vi "Add Signal.vi"(8 "error in":errorcluster, 9 "Signal":refnum<class "CAN Signal.lvclass">, 10 "Signal Name":string, 11 "CAN Frame in":refnum<class "CAN Frame.lvclass">) -> (0 "error out":errorcluster, 3 "CAN Frame out":refnum<class "CAN Frame.lvclass">)   [LabVIEW 2023, in "CAN Frame.lvclass"]
uses:
  CAN Frame.lvclass
  CAN Frame.lvclass/CAN Frame.ctl
  CAN Signal/CAN Signal.lvclass
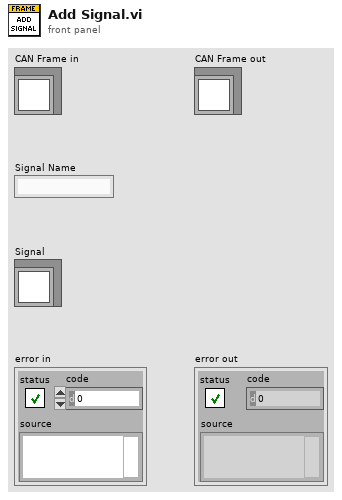
[diagram p1: front panel]
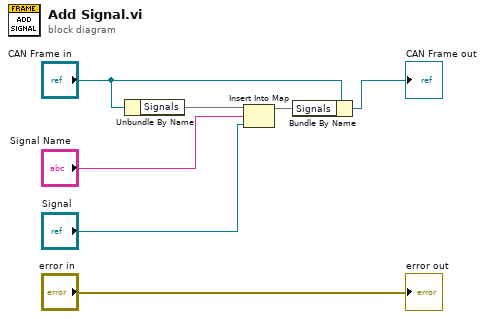
[diagram p0: block diagram]
diagram:
  n1 = Unbundle By Name("CAN Frame in") -> ("Signals"=w6:map{string, refnum<class "CAN Signal.lvclass">})
  n2 = Insert Into Map(map in=w6, key="Signal Name", value="Signal") -> (map out=w3:map{string, refnum<class "CAN Signal.lvclass">})  [unwired: 2 out]
  n3 = Bundle By Name(cluster="CAN Frame in", "Signals"=w3) -> (→"CAN Frame out":refnum<class "CAN Frame.lvclass">)
  "error out" <- "error in"
